vi "Confocal_VerTDVg.vi"() -> ()   [LabVIEW 2009]
uses:
  <vilib>/DAQmx/configure/timing.llb/DAQmx Timing (Sample Clock).vi
  <vilib>/DAQmx/create/channels.llb/DAQmx Create Channel (AI-Voltage-Basic).vi
  <vilib>/DAQmx/create/channels.llb/DAQmx Create Channel (AO-Voltage-Basic).vi
  <vilib>/DAQmx/write.llb/DAQmx Write (Analog 2D DBL NChan NSamp).vi
  <vilib>/DAQmx/read.llb/DAQmx Read (Analog 1D DBL NChan 1Samp).vi
  <vilib>/DAQmx/configure/trigger.llb/DAQmx Start Trigger (Digital Edge).vi
  <vilib>/DAQmx/read.llb/DAQmx Read (Analog 2D DBL NChan NSamp).vi
  <vilib>/DAQmx/write.llb/DAQmx Write (Analog 1D DBL NChan 1Samp).vi
  <vilib>/measure/NI_MABase.lvlib
  Program Files (x86)/National Instruments/LabVIEW 2009/resource/objmgr/daqmx.rc
panel:
  out "Boolean":bool=TRUE
  in  "Update":bool
  in  "StopPoint":dbl
  in  "Concat":bool
  in  "Increment":bool
  in  "stepsize":dbl=0.001
  in  "y 2":cluster{dbl, string, tag}[](array[cluster])=[{1.0, "", "Dev1/ai18"}, {1.0, "", "Dev1/ai16"}, {1.0, "", ""}, {1.0, "", ""}, {0.0, "", ""}, {1.0, "", ""}]
  in  "y":cluster{dbl, string, tag}[](array[cluster])=[{1.0, "", "Dev1/ao1"}, {1.0, "", "Dev1/ao0"}, {1.0, "", "Dev1/ao2"}, {1.0, "", "Dev1/ao3"}, {0.0, "", ""}, {1.0, "", ""}]
  in  "?":bool
  in  "Output4":dbl min=-10.0 max=10.0 step=0.1
  in  "Output3":dbl min=-10.0 max=10.0 step=0.1
  in  "Starting Point for Scan":tag="Dev1/ai1:2"
  in  "output scale":i32=1
  in  "out/in":dbl=1.0
  in  "Channel 2":path=path "C:/Users/debordet/Desktop/Physics Research/CNT PGM/Data/Scans/2011-10-7/J15_[16]_PA1"
  in  "Channel 1":path=path "C:/Users/debordet/Desktop/Physics Research/CNT PGM/Data/Scans/2011-10-7/J15_[16]_Refl1"
  in  "Save Image":bool
  out "Channel2":dbl[][](graph)
  in  "Scanner delay (ms)":dbl=0.16
  in  "Lines read":u32=1
  out "Reflection Image":dbl[][](graph)
  out "Linescan":dbl[][](graph)=[[0.06856738193309811, 0.06824489935784073, 0.06727745163238377, 0.06727745163238377, 0.06792241678263589, 0.06792241678263589, 0.06759993420748357, 0.06792241678263589, 0.06792241678263589, 0.06759993420748357, 0.06792241678263589, 0.06792241678263589, 0.06856738193309811, 0.06792241678263589, 0.06759993420748357, 0.06824489935784073, 0.06759993420748357, 0.06759993420748357, 0.06727745163238377, 0.06727745163238377, 0.06759993420748357, 0.06695496905733647, 0.06759993420748357, 0.06759993420748357, 0.06727745163238377, 0.06856738193309811, 0.06824489935784073, 0.06792241678263589, 0.06792241678263589, 0.06856738193309811, 0.06856738193309811, 0.06856738193309811, 0.06888986450840807, 0.06921234708377061, 0.06985731223465351, 0.06985731223465351, 0.07050227738574695, 0.07050227738574695, 0.07082475996137268, 0.0711472425370511, 0.07146972511278223, 0.07146972511278223, 0.0711472425370511, 0.0711472425370511, 0.07082475996137268, 0.06985731223465351, 0.06985731223465351, 0.06985731223465351, 0.06888986450840807, 0.06824489935784073, 0.06759993420748357, 0.06759993420748357, 0.06727745163238377, 0.06727745163238377, 0.06695496905733647, 0.06695496905733647, 0.06663248648234164, 0.06727745163238377, 0.06695496905733647, 0.06727745163238377, 0.06759993420748357, 0.06759993420748357, 0.06792241678263589, 0.06759993420748357, 0.06856738193309811, 0.06856738193309811, 0.06888986450840807, 0.06792241678263589, 0.06824489935784073, 0.06759993420748357, 0.06792241678263589, 0.06727745163238377, 0.06759993420748357, 0.06695496905733647, 0.06727745163238377, 0.06695496905733647, 0.06663248648234164, 0.06663248648234164, 0.06663248648234164, 0.06631000390739929, 0.06631000390739929, 0.06631000390739929, 0.06631000390739929, 0.06598752133250936, 0.06598752133250936, 0.06566503875767186, 0.06598752133250936, 0.06631000390739929, 0.06598752133250936, 0.06631000390739929, 0.06598752133250936, 0.06534255618288677, 0.06566503875767186, 0.06469759103347372, 0.06437510845884574, 0.06244021301217625, 0.05857042212447406, 0.04825097979380309, 0.04276877607709824, 0.03599664209450654, 0.029546990703332412, 0.025032234741517494, 0.02438726960491914, 0.025677199878316508, 0.02761209528991893, 0.03341678153560791, 0.0401889155096509, 0.04760601464989135, 0.05470063124426199, 0.05953786984569621, 0.062117730437914236, 0.06179524786370443, 0.06308517816085697, 0.06308517816085697, 0.06405262588427009, 0.06502007360815405, 0.06534255618288677, 0.06598752133250936, 0.06534255618288677, 0.06405262588427009, 0.06276269558649049, 0.05953786984569621, 0.05695800925681054, 0.05534559639044516, 0.05405566609828603, 0.05470063124426199, 0.05566807896361449, 0.05502311381732767, 0.053410700952517126, 0.05212077066159994, 0.04857346236583612, 0.04502615407629937, 0.04341374121947115, 0.040511398080403126, 0.040511398080403126, 0.040511398080403126, 0.04147884579296599, 0.0418013283639224, 0.0421238109349299, 0.04276877607709824, 0.0418013283639224, 0.0401889155096509, 0.03760905494546761, 0.03470671181465164, 0.03244933382685677, 0.03180436868794224, 0.03244933382685677, 0.03502919438453927, 0.039221467797700145, 0.04147884579296599, 0.0456711192193894, 0.04792849722182151, 0.04825097979380309, 0.0456711192193894, 0.042446293505988504, 0.03631912466459714, 0.03277181639638989, 0.025032234741517494, 0.02180740906052947, 0.020839961357208617, 0.022129891628403037, 0.02535471730989191, 0.029869473272411, 0.03857650265665441, 0.0456711192193894, 0.05276573580695514, 0.057602974403720045, 0.06115028271544139, 0.06308517816085697, 0.06405262588427009, 0.06598752133250936, 0.06663248648234164, 0.06727745163238377, 0.06727745163238377, 0.06695496905733647, 0.06598752133250936, 0.06534255618288677, 0.06469759103347372, 0.06437510845884574, 0.06373014330974676, 0.06469759103347372, 0.06502007360815405, 0.06566503875767186, 0.06598752133250936, 0.06631000390739929, 0.06566503875767186, 0.06663248648234164, 0.06566503875767186, 0.06534255618288677, 0.06469759103347372, 0.06373014330974676, 0.062117730437914236, 0.060182834993437954, 0.05792545697725274, 0.057602974403720045, 0.056313044110108734, 0.05502311381732767, 0.056313044110108734, 0.05663552668343368, 0.05889290469816274], [0.014390310013197828, 0.01277789718029931, 0.01277789718029931, 0.018260100817215456, 0.017937618249940557, 0.014390310013197828, 0.02180740906052947, 0.02180740906052947, 0.019550031086813136, 0.015035275146704158, 0.021162443924932276, 0.016002722847335796, 0.006328245861055242, 0.011487966914871401, 0.005038315599569377, 0.004070867903970193, 0.013100379746779965, 0.00858562382054782, 0.008908106386386505, 0.012132932047486448, 0.02341982190039753, 0.013745344879889812, 0.03599664209450654, 0.012455414613868144, 0.018582583384540143, 0.01277789718029931, 0.05018587522677358, 0.018582583384540143, 0.018260100817215456, 0.019550031086813136, 0.01406782744651904, 0.01632520541431232, 0.00858562382054782, 0.011487966914871401, 0.008908106386386505, 0.01019803665023418, 0.013745344879889812, 0.01632520541431232, 0.008263141254758391, 0.008263141254758391, 0.008263141254758391, 0.006328245861055242, 0.011487966914871401, 0.015357757713531733, 0.01632520541431232, 0.014390310013197828, 0.021162443924932276, 0.016002722847335796, 0.021484926492705888, 0.013422862313310125, 0.022129891628403037, 0.021162443924932276, 0.016970170548414435, 0.018582583384540143, 0.022774856764300203, 0.016970170548414435, 0.018260100817215456, 0.018582583384540143, 0.01632520541431232, 0.010520519216319421, 0.007295693557685477, 0.00955307151821172, -0.00012140543853553054, 0.004393350469120888, 0.0008460422551557815, 0.006973210992092902, 0.0027809376438573193, 0.007295693557685477, 0.010843001782454027, 0.005683280730214114, 0.022129891628403037, 0.016002722847335796, 0.013745344879889812, 0.026644647583891578, 0.01632520541431232, 0.01277789718029931, 0.009875554084198285, 0.0034259027738158094, 0.009230588952274466, 0.0011685248198171903, 0.014390310013197828, 0.012455414613868144, 0.025677199878316508, 0.019227548519338968, 0.02761209528991893, 0.028257060427522004, -0.01140829516595663, 0.0237423044685213, 0.0421238109349299, 0.014712792579926194, 0.0011685248198171903, 0.02309733933232384, 0.013100379746779965, 0.010520519216319421, 0.0005235596905432037, 0.004393350469120888, 0.007618176123327238, 0.017292653115540065, 0.02309733933232384, 0.018905065951914643, 0.017937618249940557, 0.012455414613868144, 0.013100379746779965, 0.00955307151821172, 0.016002722847335796, 0.017937618249940557, 0.01987251365433717, 0.012132932047486448, 0.01632520541431232, 0.013745344879889812, 0.017292653115540065, 0.013422862313310125, 0.017615135682715433, 0.016647687981338526, 0.018260100817215456, 0.02341982190039753, 0.020839961357208617, 0.024064787036695165, 0.026967130152517085, 0.025032234741517494, 0.02535471730989191, 0.02890202556532645, 0.026644647583891578, 0.02245237419632661, 0.017292653115540065, 0.02341982190039753, 0.02051747878953489, 0.015035275146704158, 0.014712792579926194, 0.012132932047486448, 0.00955307151821172, 0.006650728426549496, 0.01406782744651904, 0.00471583303432061, 0.013100379746779965, 0.01406782744651904, 0.010843001782454027, 0.014712792579926194, 0.019550031086813136, 0.014390310013197828, 0.017292653115540065, 0.013100379746779965, 0.016002722847335796, 0.006650728426549496, 0.011810449481154207, 0.019550031086813136, 0.004393350469120888, 0.017615135682715433, 0.014712792579926194, 0.04696104950618525, 0.016002722847335796, 0.04147884579296599, 0.013745344879889812, 0.011165484348638014, 0.005038315599569377, 0.011165484348638014, 0.015035275146704158, 0.026322165015316323, 0.021162443924932276, 0.01632520541431232, 0.007940658689018203, 0.005038315599569377, 0.013745344879889812, 0.016647687981338526, 0.022129891628403037, 0.02341982190039753, 0.01987251365433717, 0.017615135682715433, 0.010520519216319421, 0.012132932047486448, 0.011165484348638014, 0.00955307151821172, 0.01632520541431232, 0.012132932047486448, 0.007618176123327238, 0.01406782744651904, 0.009875554084198285, 0.01019803665023418, 0.007618176123327238, 0.013100379746779965, 0.010520519216319421, 0.006328245861055242, 0.013745344879889812, 0.006328245861055242, 0.008908106386386505, 0.015035275146704158, 0.013100379746779965, 0.019550031086813136, 0.014712792579926194, 0.018582583384540143, 0.01987251365433717, 0.011810449481154207, 0.013100379746779965, 0.015035275146704158, 0.017615135682715433, 0.010843001782454027, 0.00858562382054782, 0.006973210992092902, 0.01019803665023418, 0.007618176123327238]]
  out "Output rate":dbl=31250.0
  out "Input rate":dbl=31250.0
  in  "Y Scan size(um)":dbl=3.0
  in  "Reset":bool
  in  "Stop":bool
  in  "Continuous \nScan":bool=TRUE
  in  "Finite scan":bool
  in  "Conversion \n(mV/um)":dbl=41.0
  in  "Scan Lines":u32=200
  in  "Scan Points":u32=200
  in  "Scan Angle (degrees)":dbl
  in  "X offset (um)":dbl
  in  "Y offset (um)":dbl
  in  "Scan Rate (Hz)":dbl=25.0
  in  "X Scan size(um)":dbl=3.0
  in  "minimum value":dbl=-4.0 caption="Output Minimum Value" format="%0.2f"
  in  "maximum value":dbl=4.0 caption="Output Maximum Value" format="%0.2f"
  in  "Maximum Value":dbl=10.0 caption="Input Maximum Value" format="%0.2f"
  in  "Minimum Value":dbl=-10.0 caption="Input Minimum Value" format="%0.2f"
  # "Scan channel 1"
  # "Scan channel 2"
  # "Device"
  # "Output channel 3"
  # "Output channel 4"
  # "Input channel 1"
  # "Input channel 2"
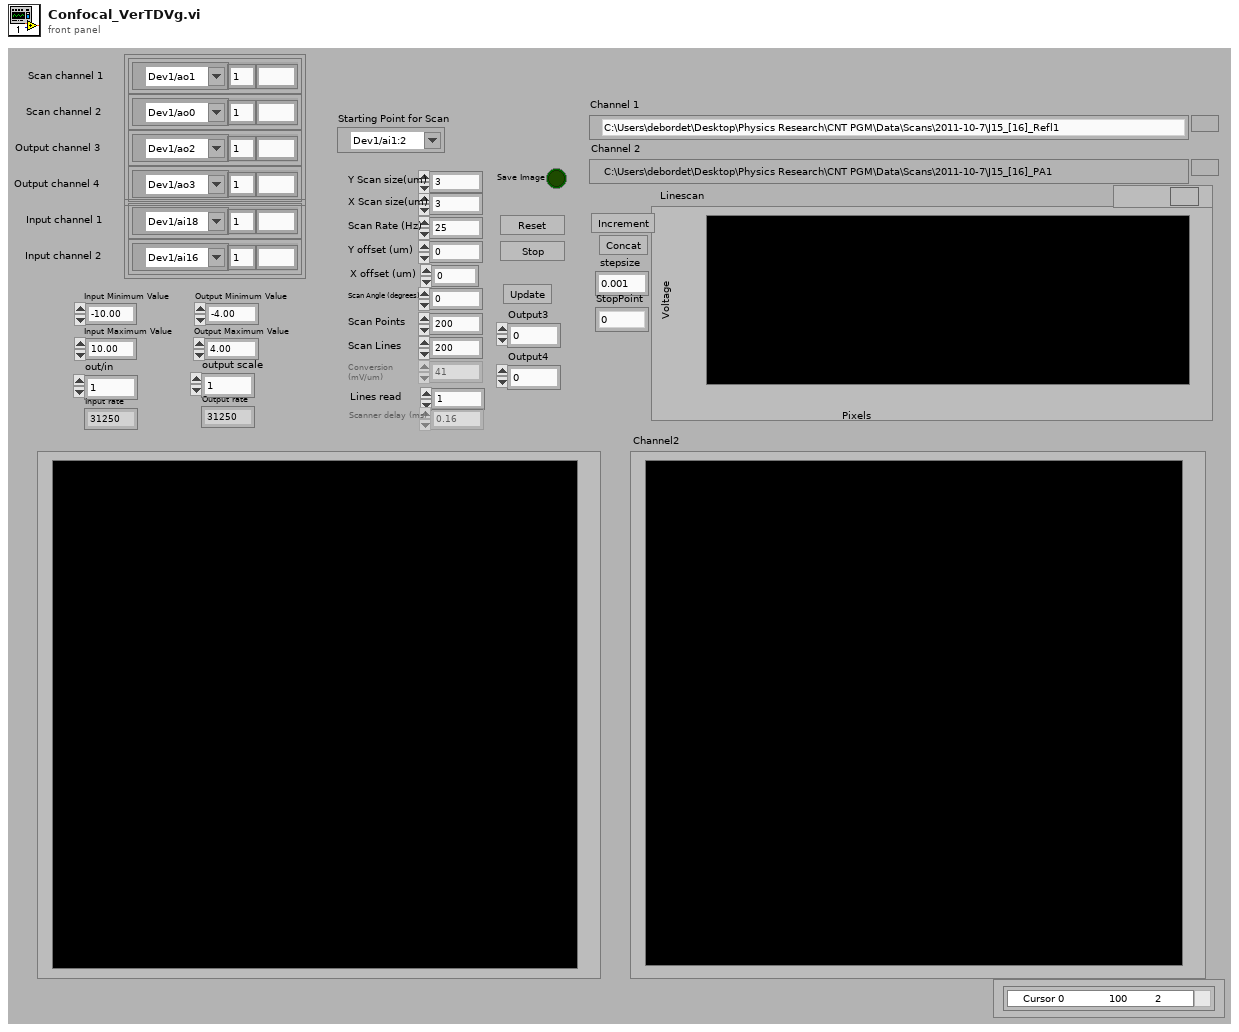
[diagram p1: front panel]
types:
  T1 = enum16{"Sine Wave", "Triangle Wave", "Square Wave", "Sawtooth Wave"}
  T2 = cluster{"Y Scan size(um) ":dbl, "X Scan size(um)":dbl, "Scan Rate (Hz)":dbl, "Y offset (um)":dbl, "X offset (um)":dbl, "Scan Angle (degrees)":dbl, "Scan Points":u32, "Scan Lines":u32, "Conversion \n(mV/um)":dbl, "Finite scan":bool, "Continuous \nScan":bool, "Lines read":u32, "Scanner delay (ms)":dbl}
  T3 = enum16{"open", "open or create", "create or replace", "create", "open (read only)"}
  T4 = typedef "LVPointDoubleTypeDef.ctl" = cluster{"Cursor X":dbl, "Cursor Y":dbl}
  T5 = cluster{"X offset (um)":dbl, "Y offset (um)":dbl}
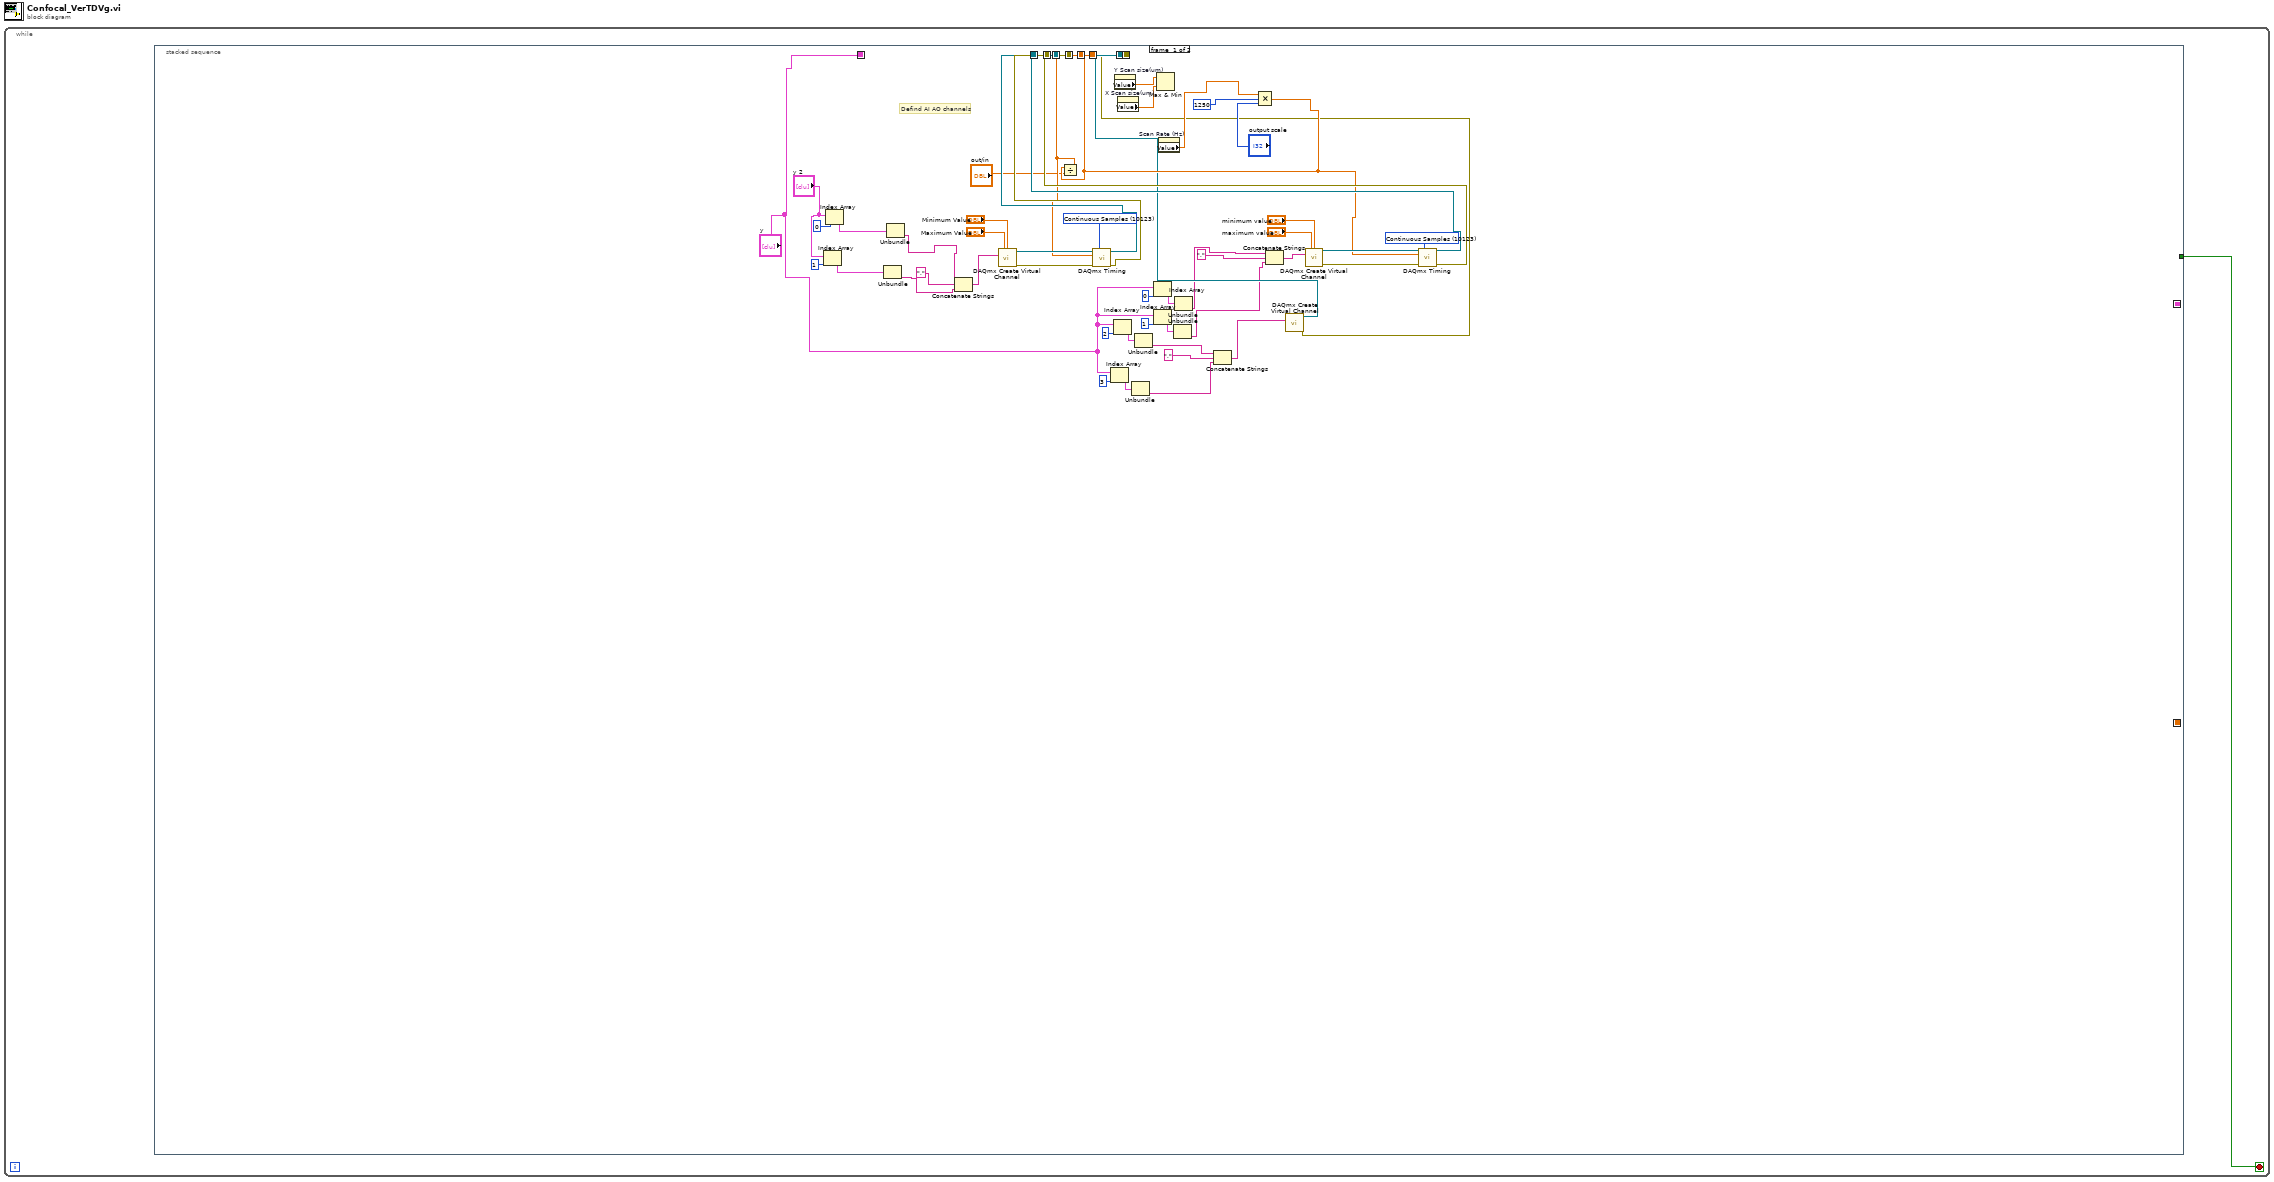
[diagram p0: block diagram]
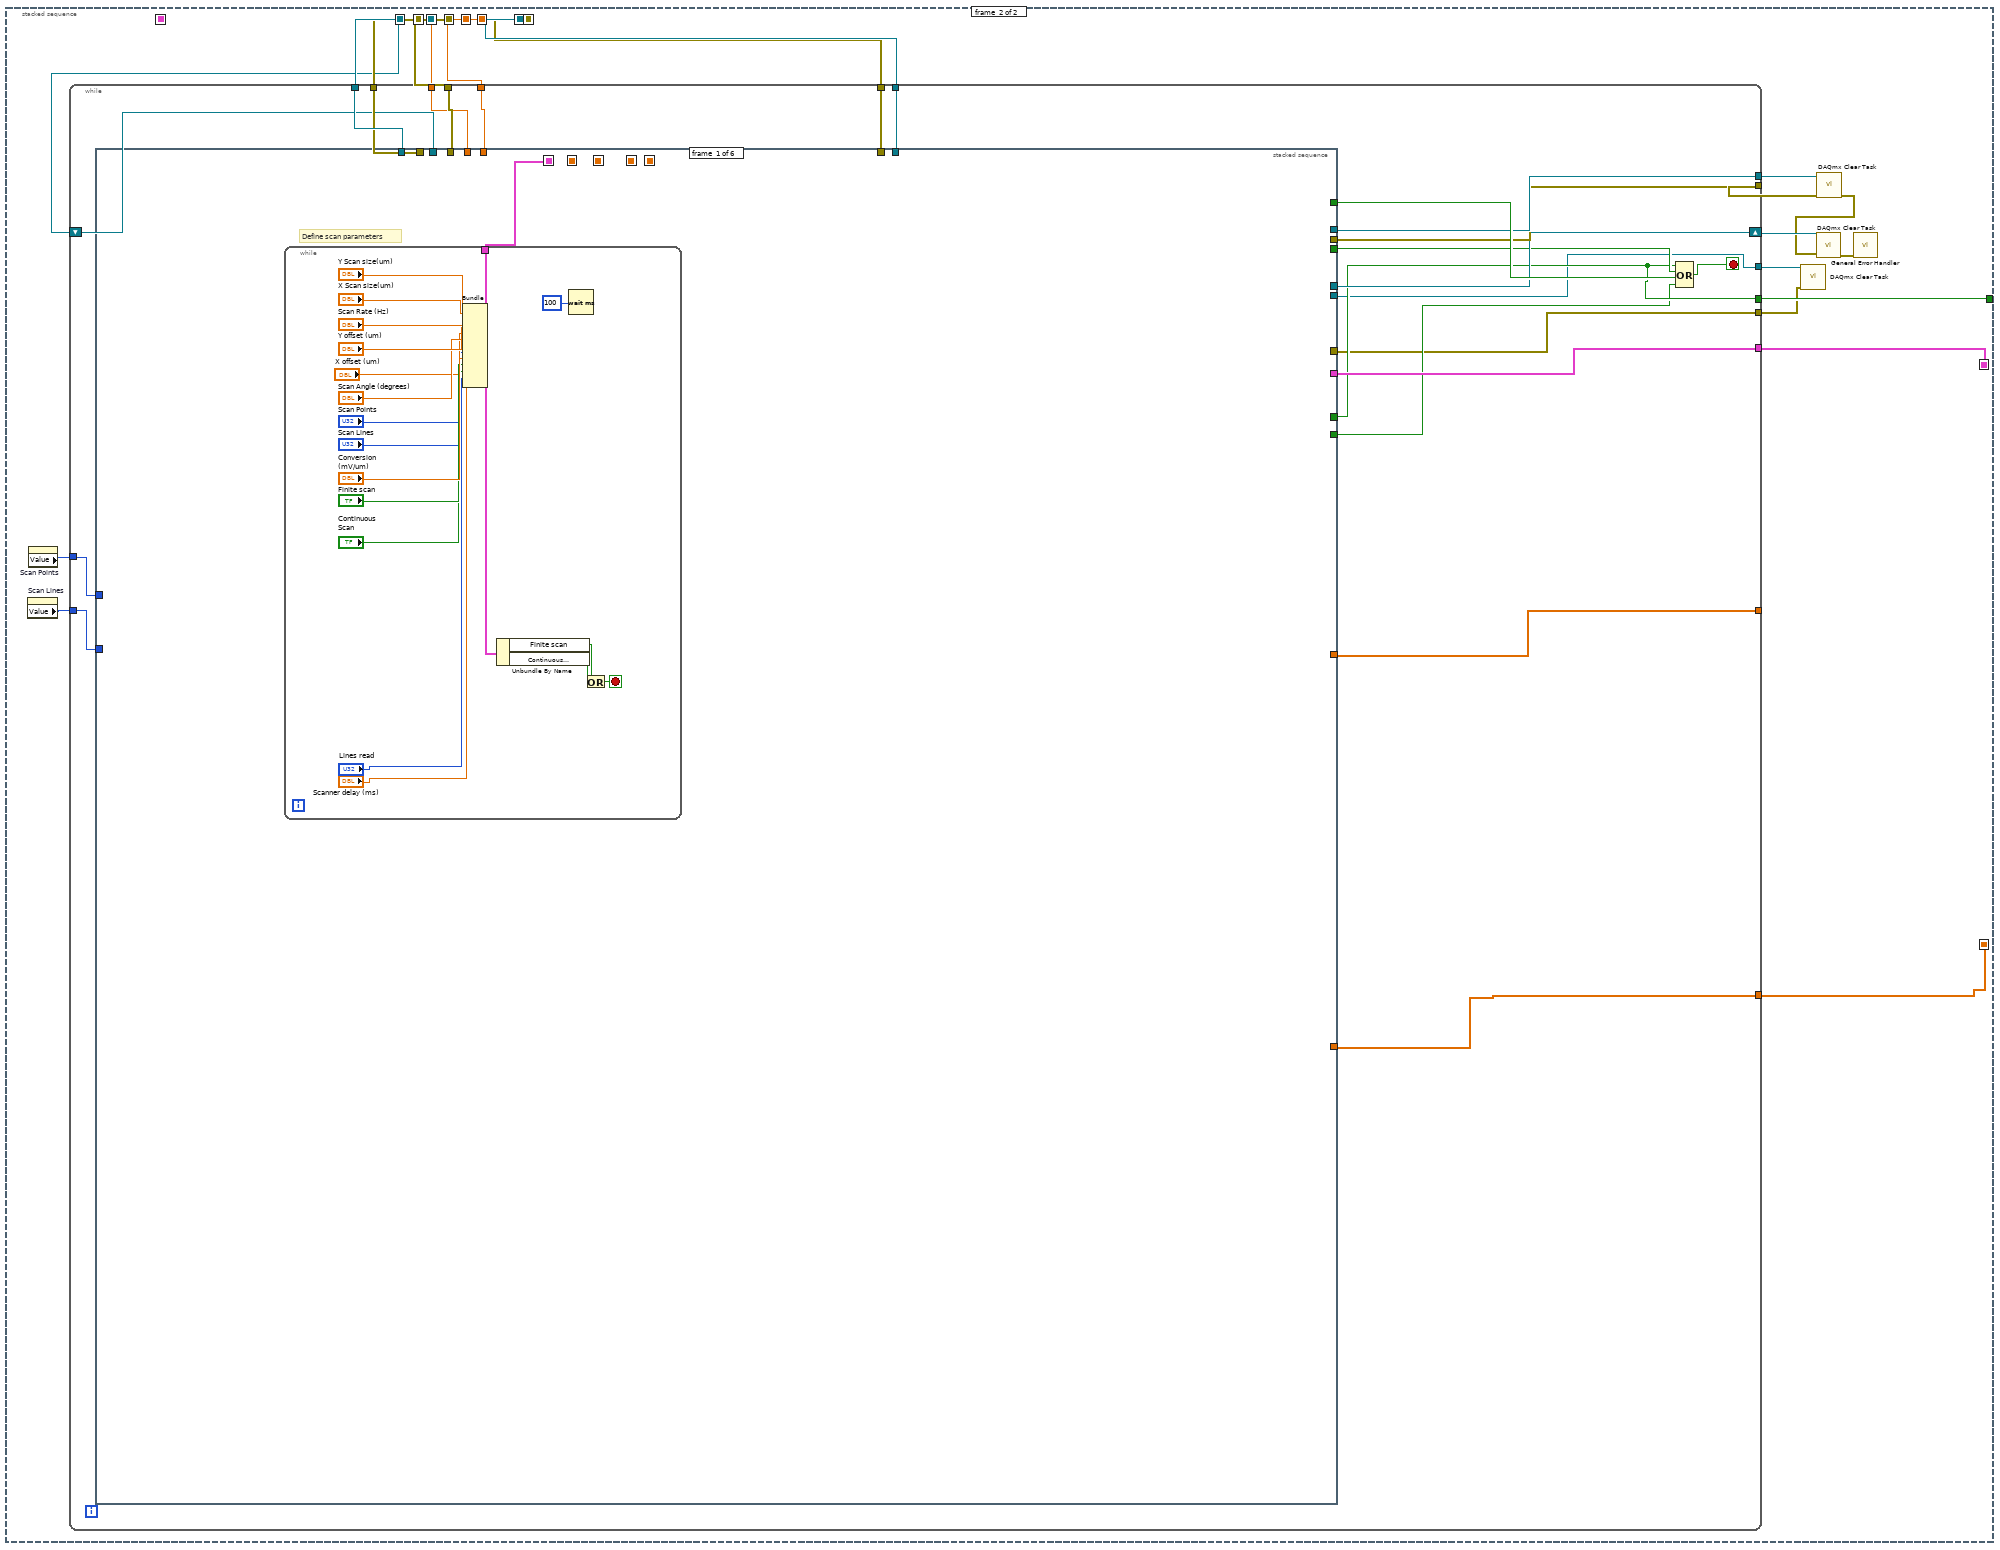
[diagram p2: hidden frame]
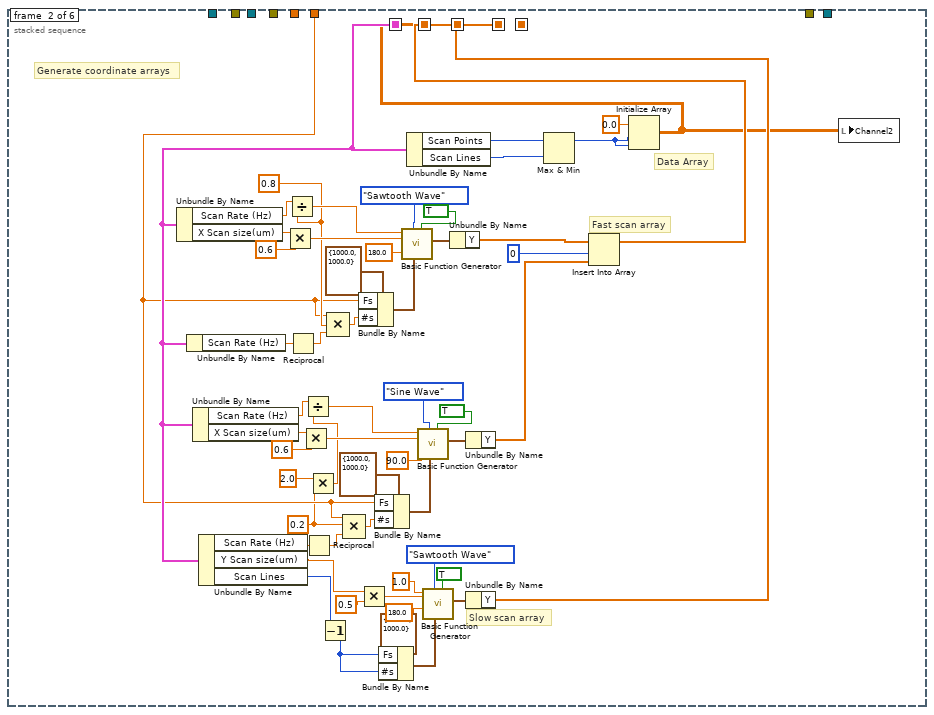
[diagram p3: hidden frame]
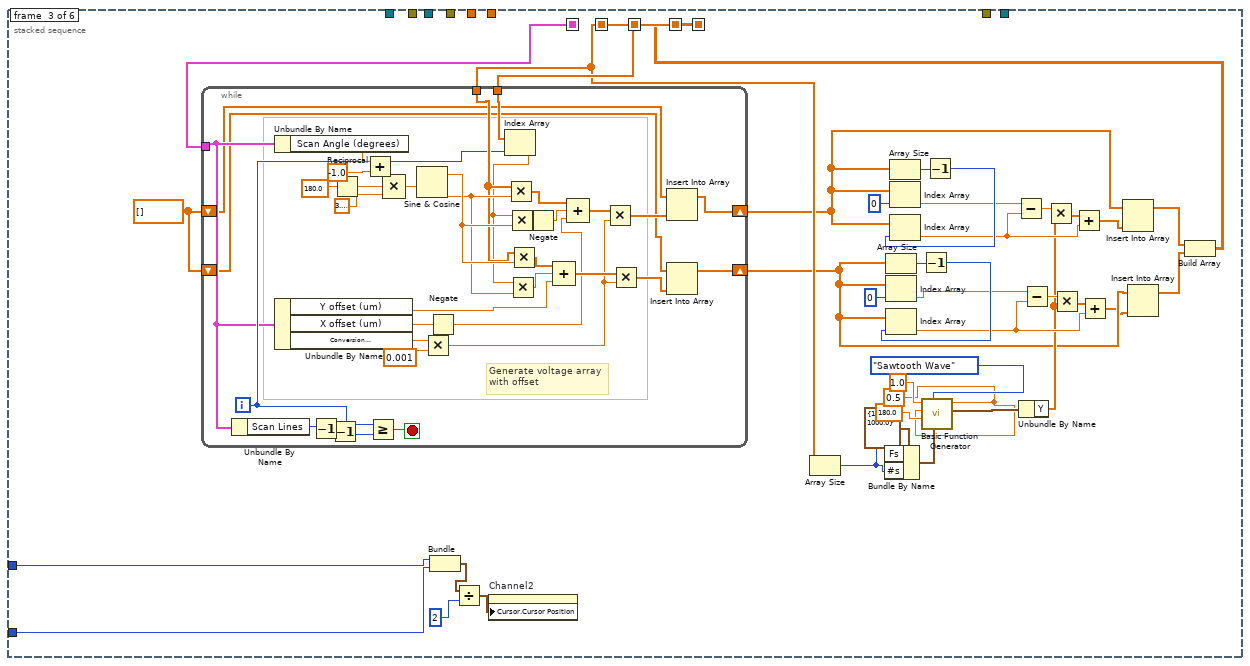
[diagram p4: hidden frame]
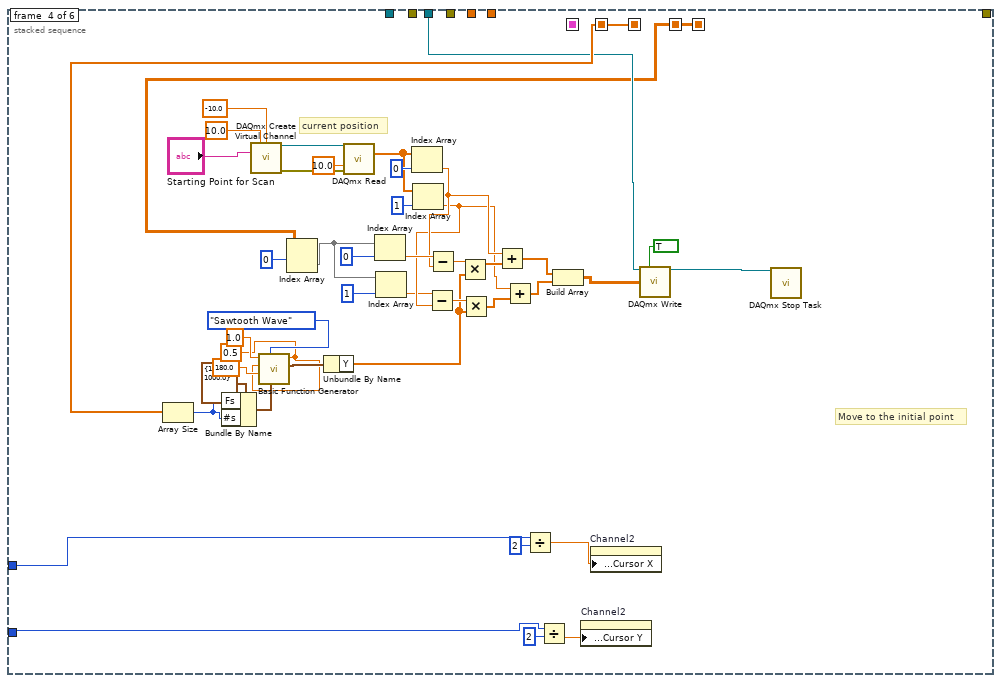
[diagram p5: hidden frame]
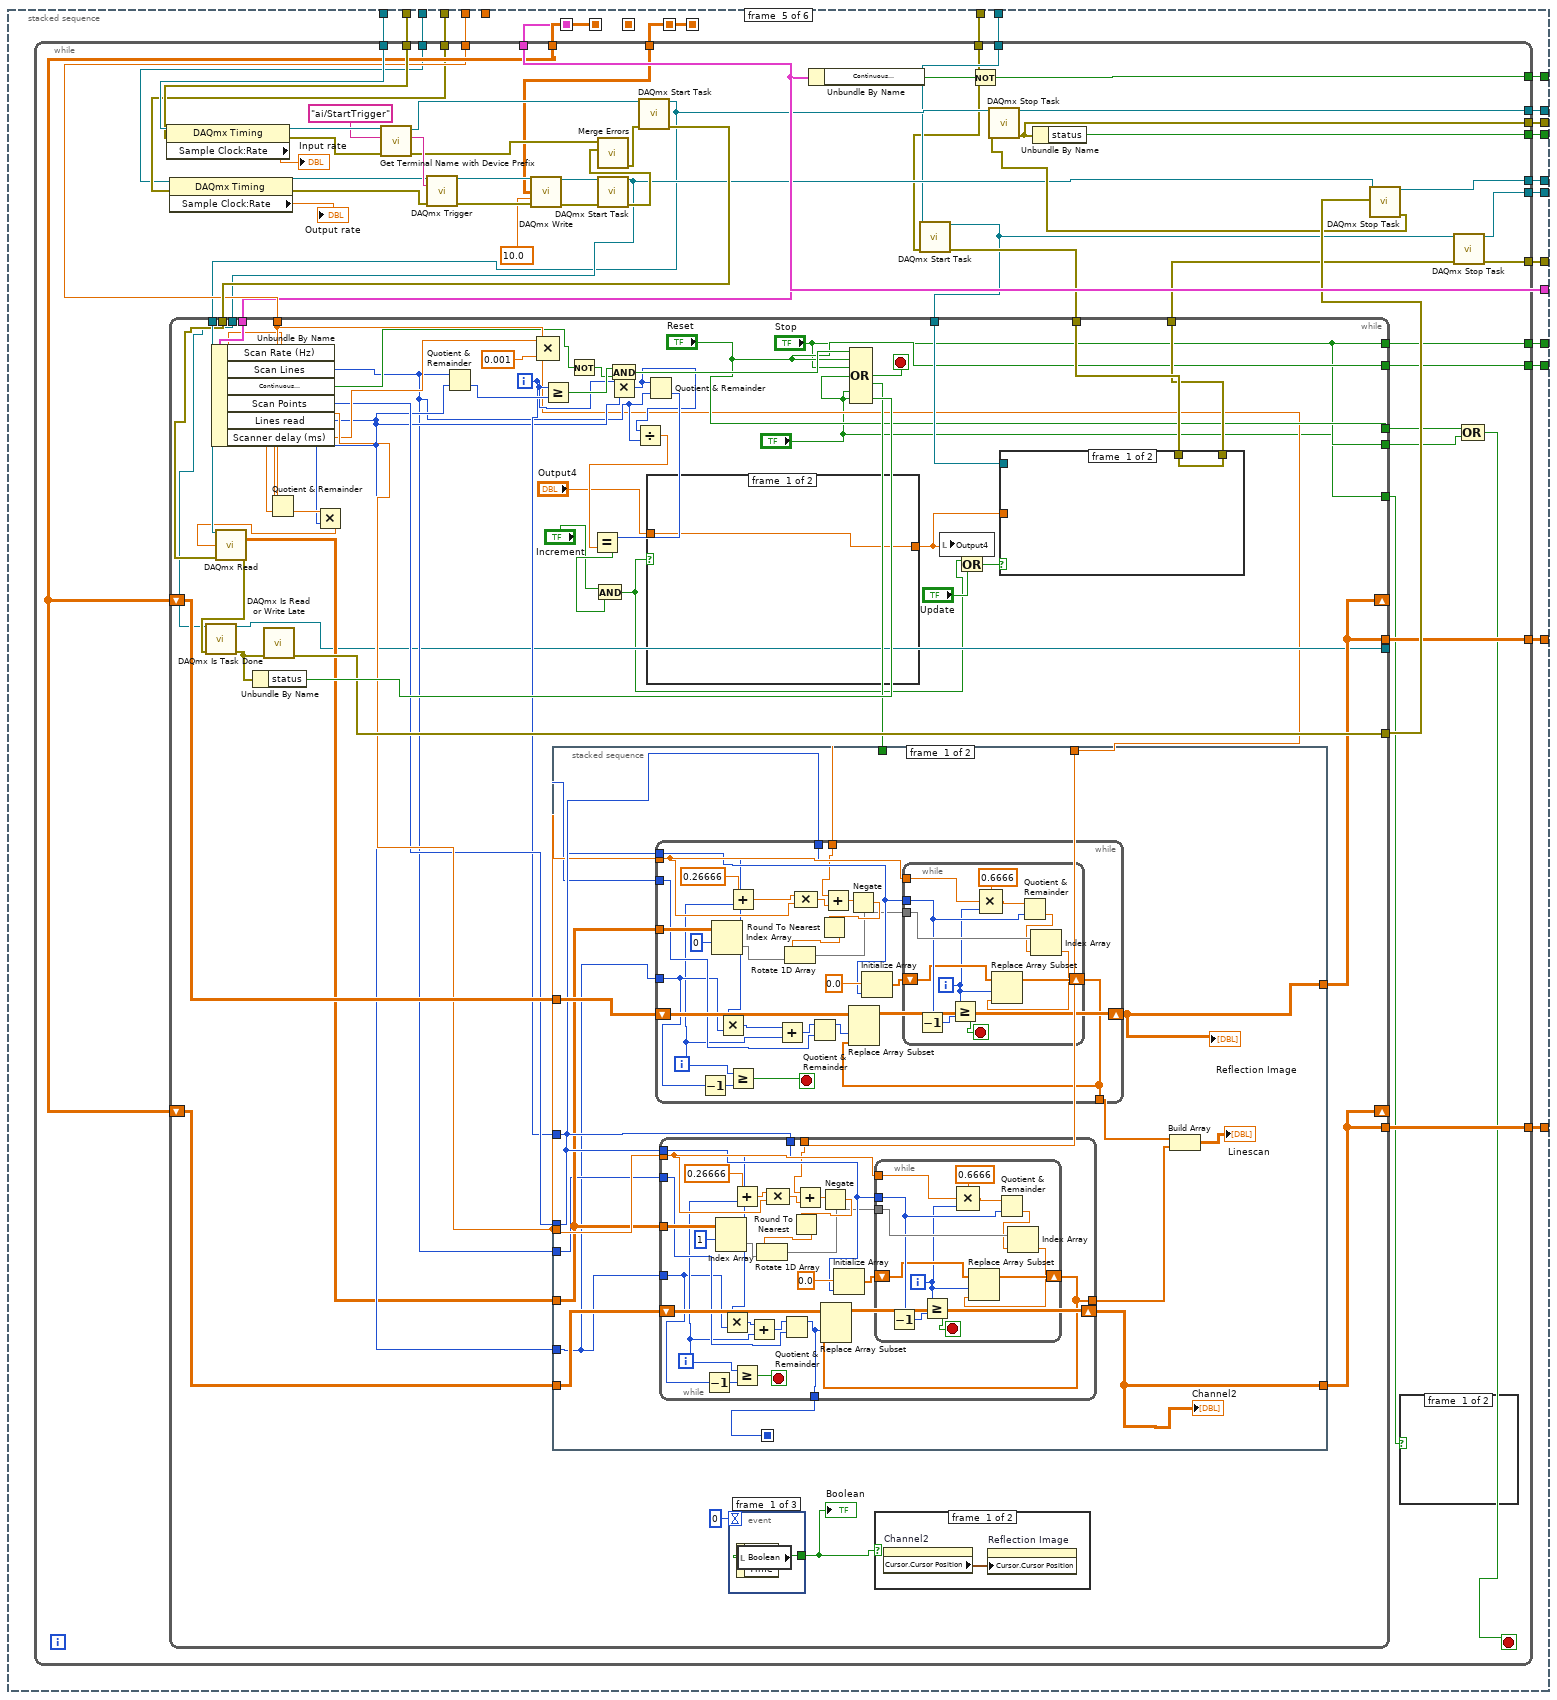
[diagram p6: hidden frame]
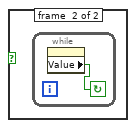
[diagram p7: hidden frame]
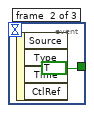
[diagram p8: hidden frame]
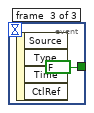
[diagram p9: hidden frame]
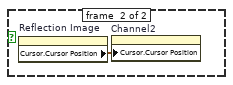
[diagram p10: hidden frame]
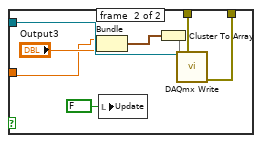
[diagram p11: hidden frame]
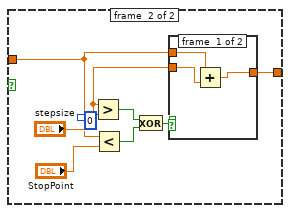
[diagram p12: hidden frame]
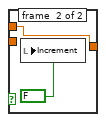
[diagram p13: hidden frame]
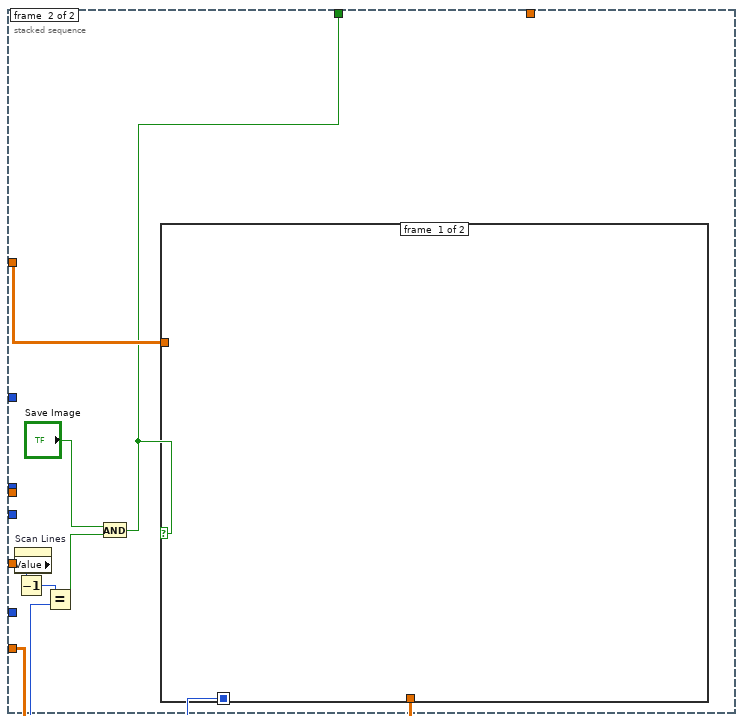
[diagram p14: hidden frame]
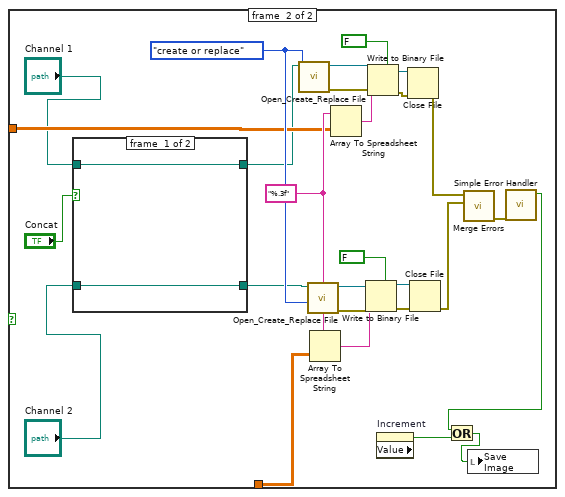
[diagram p15: hidden frame]
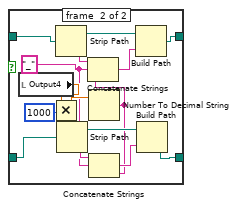
[diagram p16: hidden frame]
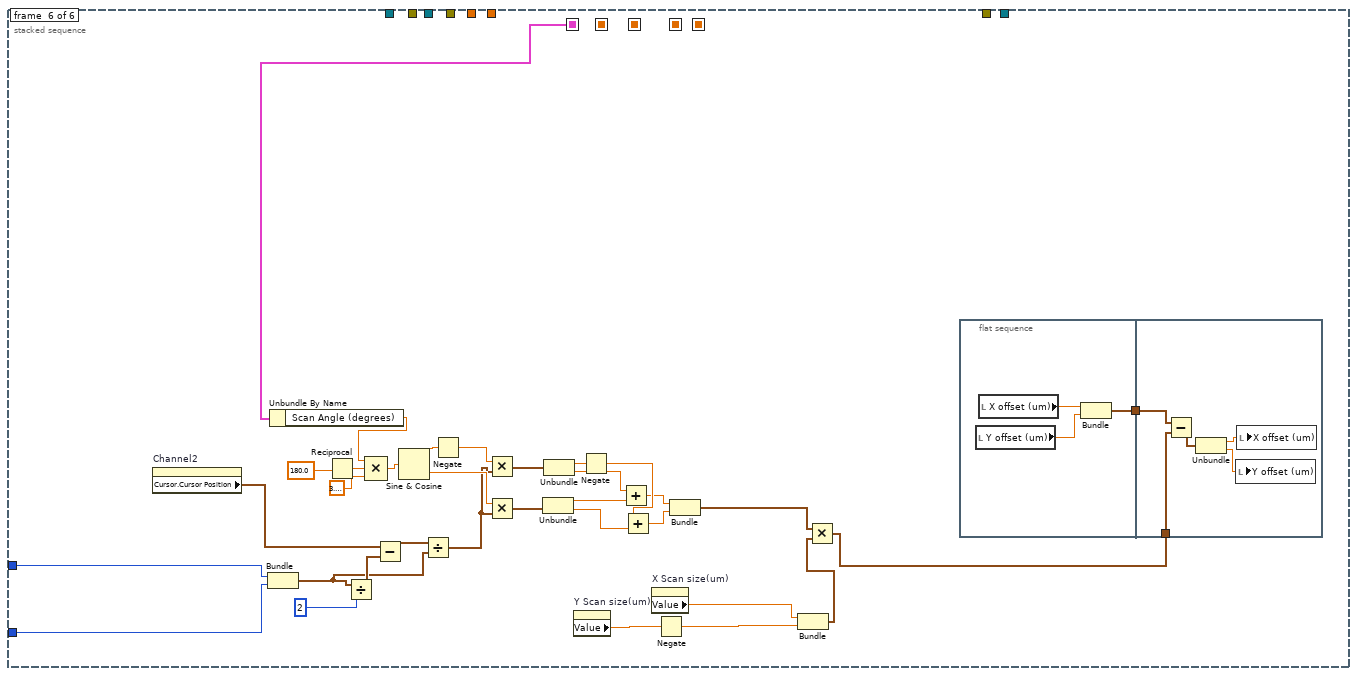
[diagram p17: hidden frame]
diagram:
  n1 = while {
    stop <- w1 stop-if-true
    n2 = stacked-sequence {
      seq-local: [w39 _] -> [_ w70]
      seq-local: [w42 _] -> [_ w69]
      seq-local: [w41 _] -> [_ w62]
      seq-local: [w40 _] -> [_ w68]
      seq-local: [w34 _] -> [_ w67]
      seq-local: [w33 _] -> [_ w71]
      seq-local: [_ w61] -> [_ _]
      seq-local: [_ w60] -> [_ _]
      seq-local: [w29 _] -> [_ w56]
      seq-local: [w28 _] -> [_ w55]
      seq-local: ["y" _] -> [_ _]
      tunnel: [_ w57] -> w1
      frame #0 {
        w44 = 10123 items=["Finite Samples"=10178, "Continuous Samples"=10123] ("sample mode")
        w49 = 10123 items=["Finite Samples"=10178, "Continuous Samples"=10123] ("sample mode")
        # "Defind AI AO channels"
        n3 = Index Array(array="y 2", index=1) -> (element=w20:cluster{dbl, string, tag})
        n4 = Index Array(array="y 2", index=0) -> (element=w22:cluster{dbl, string, tag})
        n5 = Unbundle(w20) -> (w2:tag)  [unwired: 2 out]
        n6 = Unbundle(w22) -> (w3:tag)  [unwired: 2 out]
        n7 = Concatenate Strings(w3, ",", w2) -> (w27:string)
        n8 = call-poly <vilib>:"DAQmx Create Virtual Channel.vi"("maximum value"="Maximum Value", "minimum value"="Minimum Value", "physical channels"=w27) -> ("task out"=w47:refnum<k21>, "error out"=w48:errorcluster)  [unwired: 11 in]
        n9 = Index Array(array="y", index=3) -> (element=w15:cluster{dbl, string, tag})
        n10 = Index Array(array="y", index=2) -> (element=w17:cluster{dbl, string, tag})
        n11 = property on="Y Scan size(um)" class="Digital (strict)"() -> ("Value"=w36:dbl)  [unwired: 2 in, 2 out]
        n12 = property on="X Scan size(um)" class="Digital (strict)"() -> ("Value"=w35:dbl)  [unwired: 2 in, 2 out]
        n13 = Unbundle(w15) -> (w13:tag)  [unwired: 2 out]
        n14 = Unbundle(w17) -> (w14:tag)  [unwired: 2 out]
        n15 = Index Array(array="y", index=1) -> (element=w9:cluster{dbl, string, tag})
        n16 = Index Array(array="y", index=0) -> (element=w11:cluster{dbl, string, tag})
        n17 = Max & Min(x=w36, y=w35) -> ()  [unwired: 2 out]
        n18 = property on="Scan Rate (Hz)" class="Digital (strict)"() -> ("Value"=w31:dbl)  [unwired: 2 in, 2 out]
        n19 = Unbundle(w9) -> (w7:tag)  [unwired: 2 out]
        n20 = Unbundle(w11) -> (w8:tag)  [unwired: 2 out]
        n21 = Concatenate Strings(w14, ",", w13) -> (w4:string)
        n22 = Compound Arithmetic op=MULTIPLY(w31, 1250, "output scale") -> (w33:dbl)
        n23 = Divide(x=w33, y="out/in") -> (x/y=w34:dbl)
        n24 = call-poly <vilib>:"DAQmx Timing.vi"("task/channels in"=w47, "sample mode"=w49, "rate"=w34, "error in"=w48) -> ("task out"=w39:refnum<k21>, "error out"=w42:errorcluster)  [unwired: 10 in]
        n25 = Concatenate Strings(w8, ",", w7) -> (w24:string)
        n26 = call-poly <vilib>:"DAQmx Create Virtual Channel.vi"("physical channels"=w4) -> ("task out"=w29:refnum<k21>, "error out"=w28:errorcluster)  [unwired: 13 in]
        n27 = call-poly <vilib>:"DAQmx Create Virtual Channel.vi"("maximum value"="maximum value", "minimum value"="minimum value", "physical channels"=w24) -> ("task out"=w38:refnum<k21>, "error out"=w43:errorcluster)  [unwired: 11 in]
        n28 = call-poly <vilib>:"DAQmx Timing.vi"("task/channels in"=w38, "sample mode"=w44, "rate"=w33, "error in"=w43) -> ("task out"=w41:refnum<k21>, "error out"=w40:errorcluster)  [unwired: 10 in]
      }
      frame #1 {
        n29 = property on="Scan Lines" class="Digital (strict)"() -> ("Value"=w59:u32)  [unwired: 2 in, 2 out]
        n30 = property on="Scan Points" class="Digital (strict)"() -> ("Value"=w58:u32)  [unwired: 2 in, 2 out]
        n31 = while {
          tunnel: w71 -> [w94]
          tunnel: w70 -> [w93]
          tunnel: w69 -> [w92]
          tunnel: w68 -> [w91]
          tunnel: w67 -> [w90]
          tunnel: [w88] -> w66
          tunnel: [w87] -> w65
          shift-right: [w85] -> w64
          shift-left: w62 -> [w84]
          tunnel: [w83] -> _
          tunnel: [w82] -> w61
          tunnel: [w80] -> w60
          tunnel: w59 -> [w79]
          tunnel: w58 -> [w78]
          tunnel: [w77] -> w57
          tunnel: w56 -> [w75]
          tunnel: w55 -> [w74]
          tunnel: [w73] -> w53
          tunnel: [w72] -> w52
          stop <- w86 stop-if-true
          n32 = stacked-sequence {
            seq-local: [w95 _ _ _ _ _] -> [_ w139 w207 _ w295 w612]
            seq-local: [_ w114 _ _ _ _] -> [_ _ _ _ w302 _]
            seq-local: [_ w115 _ _ _ _] -> [_ _ w197 w256 _ _]
            seq-local: [_ w116 _ _ _ _] -> [_ _ w208 _ _ _]
            seq-local: [_ _ w170 _ _ _] -> [_ _ _ w252 w299 _]
            tunnel: w94 -> [_ w138 _ _ _ _]
            tunnel: w93 -> [_ _ _ _ w310 _]
            tunnel: w92 -> [_ _ _ _ w309 _]
            tunnel: w84 -> [_ _ _ w254 w298 _]
            tunnel: w91 -> [_ _ _ _ w308 _]
            tunnel: w90 -> [_ _ _ _ w300 _]
            tunnel: [_ _ _ _ w307 _] -> w77
            tunnel: [_ _ _ _ w306 _] -> w81
            tunnel: [_ _ _ _ w301 _] -> w89
            tunnel: [_ _ _ _ w305 _] -> w88
            tunnel: [_ _ _ _ w304 _] -> w87
            tunnel: [_ _ _ _ w303 _] -> w85
            tunnel: [_ _ _ _ w297 _] -> w83
            tunnel: [_ _ _ _ w296 _] -> w82
            tunnel: [_ _ _ _ w295 _] -> w80
            tunnel: [_ _ _ _ w294 _] -> w76
            tunnel: w79 -> [_ _ w172 w246 _ w587]
            tunnel: w78 -> [_ _ w173 w247 _ w586]
            tunnel: w75 -> [_ _ _ _ w293 _]
            tunnel: w74 -> [_ _ _ _ w292 _]
            tunnel: [_ _ _ _ w291 _] -> w73
            tunnel: [_ _ _ _ w290 _] -> w72
            frame #0 {
              # "Define scan parameters"
              n33 = while {
                tunnel: [w106] -> w95
                stop <- w107 stop-if-true
                n34 = Bundle("Y Scan size(um)"="Y Scan size(um)", "X Scan size(um)"="X Scan size(um)", "Scan Rate (Hz)"="Scan Rate (Hz)", "Y offset (um)"="Y offset (um)", "X offset (um)"="X offset (um)", "Scan Angle (degrees)"="Scan Angle (degrees)", "Scan Points"="Scan Points", "Scan Lines"="Scan Lines", "Conversion \n(mV/um)"="Conversion \n(mV/um)", "Finite scan"="Finite scan", "Continuous \nScan"="Continuous \nScan", "Lines read"="Lines read", "Scanner delay (ms)"="Scanner delay (ms)") -> (w106:T2)  [unwired: 1 in]
                n35 = Unbundle By Name(w106) -> ("Finite scan"=w105:bool, "Continuous \nScan"=w104:bool)
                n36 = Wait (ms)(milliseconds to wait=u32 100) -> ()  [unwired: 1 out]
                n37 = Or(x=w105, y=w104) -> (x .or. y?=w107:bool)
              }
            }
            frame #1 {
              w118 = 0.2 ("value")
              w157 = 0.8 ("y")
              # "Slow scan array"
              # "Fast scan array"
              # "Data Array"
              # "Generate coordinate arrays"
              n38 = Unbundle By Name(w139) -> ("Scan Rate (Hz)"=w162:dbl, "X Scan size(um)"=w165:dbl)
              n39 = Unbundle By Name(w139) -> ("Scan Rate (Hz)"=w155:dbl)
              n40 = Unbundle By Name(w139) -> ("Scan Rate (Hz)"=w147:dbl, "X Scan size(um)"=w150:dbl)
              n41 = Unbundle By Name(w139) -> ("Scan Rate (Hz)"=w141:dbl, "Y Scan size(um)"=w130:dbl, "Scan Lines"=w131:u32)
              n42 = Multiply(x=w165, y=0.6) -> (x*y=w163:dbl)
              n43 = Divide(x=w162, y=w157) -> (x/y=w161:dbl)
              n44 = Reciprocal(x=w155) -> (1/x=w156:dbl)
              n45 = Multiply(x=w150, y=0.6) -> (x*y=w148:dbl)
              n46 = Reciprocal(x=w141) -> (1/x=w142:dbl)
              n47 = Multiply(x=2.0, y=w118) -> (x*y=w117:dbl)
              n48 = Divide(x=w147, y=w117) -> (x/y=w146:dbl)
              n49 = Decrement(x=w131) -> (x-1=w123:u32)
              n50 = Compound Arithmetic op=MULTIPLY(w138, w157, w156) -> (w158:dbl)
              n51 = Compound Arithmetic op=MULTIPLY(w138, w118, w142) -> (w143:dbl)
              n52 = Bundle By Name(cluster=cluster{"Fs":dbl, "#s":dbl} {"Fs"=1000.0, "#s"=1000.0} ("sampling info"), "Fs"=w138, "#s"=w158) -> (w159:cluster{"Fs":dbl, "#s":dbl})
              n53 = Multiply(x=w130, y=0.5) -> (x*y=w129:dbl)
              n54 = Bundle By Name(cluster=cluster{"Fs":dbl, "#s":dbl} {"Fs"=1000.0, "#s"=1000.0} ("sampling info"), "Fs"=w138, "#s"=w143) -> (w144:cluster{"Fs":dbl, "#s":dbl})
              n55 = Bundle By Name(cluster=cluster{"Fs":dbl, "#s":dbl} {"Fs"=1000.0, "#s"=1000.0} ("sampling info"), "Fs"=w123, "#s"=w123) -> (w132:cluster{"Fs":dbl, "#s":dbl})
              n56 = call <vilib>:"Basic Function Generator.vi"("reset signal"=TRUE, "sampling info"=w159, "signal type"=T1."Sawtooth Wave", "phase"=180.0, "amplitude"=w163, "frequency"=w161) -> ("signal out"=w154:waveform(dbl))  [unwired: 3 in, 2 out]
              n57 = Unbundle By Name(w139) -> ("Scan Points"=w122:u32, "Scan Lines"=w121:u32)
              n58 = call <vilib>:"Basic Function Generator.vi"("reset signal"=TRUE, "sampling info"=w144, "signal type"=T1."Sine Wave", "phase"=90.0, "amplitude"=w148, "frequency"=w146) -> ("signal out"=w140:waveform(dbl))  [unwired: 3 in, 2 out]
              n59 = call <vilib>:"Basic Function Generator.vi"("reset signal"=TRUE, "sampling info"=w132, "signal type"=T1."Sawtooth Wave", "phase"=180.0, "amplitude"=w129, "frequency"=1.0) -> ("signal out"=w125:waveform(dbl))  [unwired: 3 in, 2 out]
              n60 = Unbundle By Name(w154) -> ("Y"=w127:dbl[])
              n61 = Unbundle By Name(w140) -> ("Y"=w137:dbl[])
              n62 = Unbundle By Name(w125) -> ("Y"=w116:dbl[])
              n63 = Max & Min(x=w122, y=w121) -> (max(x,y)=w120:u32)  [unwired: 1 out]
              n64 = Insert Into Array(array=w127, index=0, new element=w137) -> (w115:dbl[])
              n65 = Initialize Array(0.0 ("element"), w120, w120) -> (w114:dbl[][])
              n66 = local write "Channel2"(w114) -> ()
            }
            frame #2 {
              w199 = 0.5 ("offset")
              w206 = dbl[] []
              n67 = while {
                tunnel: w207 -> [w228]
                tunnel: w197 -> [w234]
                tunnel: w208 -> [w233]
                shift-right: [w220] -> w179
                shift-left: w206 -> [w219]
                shift-right: [w216] -> w180
                shift-left: w206 -> [w217]
                i -> [w231]
                stop <- w225 stop-if-true
                # "Generate voltage array\nwith offset"
                n68 = Unbundle By Name(w228) -> ("Scan Lines"=w230:u32)
                n69 = Unbundle By Name(w228) -> ("Scan Angle (degrees)"=w244:dbl)
                n70 = Unbundle By Name(w228) -> ("Y offset (um)"=w209:dbl, "X offset (um)"=w211:dbl, "Conversion \n(mV/um)"=w227:dbl)
                n71 = Decrement(x=w230) -> (x-1=w229:u32)
                n72 = Decrement(x=w229) -> (x-1=w215:u32)
                n73 = Reciprocal(x=180.0 ("value")) -> (1/x=w243:dbl)
                n74 = Add(x=w244, y=-1.0) -> (x+y=w214:dbl)
                n75 = Greater Or Equal?(x=w231, y=w215) -> (x >= y?=w225:bool)
                n76 = Compound Arithmetic op=MULTIPLY(w214, w243, 3.141592653589793) -> (w245:dbl)
                n77 = Sine & Cosine(0:w245) -> (1:w241:dbl, 2:w240:dbl)
                n78 = Multiply(x=w227, y=0.001) -> (x*y=w222:dbl)
                n79 = Negate(x=w211) -> (-x=w210:dbl)
                n80 = Index Array(array=w233, index=w231) -> (element=w232:dbl)
                n81 = Multiply(x=w234, y=w240) -> (x*y=w237:dbl[])
                n82 = Multiply(x=w232, y=w241) -> (x*y=w239:dbl)
                n83 = Multiply(x=w232, y=w240) -> (x*y=w236:dbl)
                n84 = Multiply(x=w234, y=w241) -> (x*y=w235:dbl[])
                n85 = Negate(x=w239) -> (-x=w238:dbl)
                n86 = Compound Arithmetic op=unknown(w235, w236, w209) -> (w223:dbl[])
                n87 = Compound Arithmetic op=unknown(w237, w238, w210) -> (w224:dbl[])
                n88 = Multiply(x=w224, y=w222) -> (x*y=w221:dbl[])
                n89 = Multiply(x=w223, y=w222) -> (x*y=w218:dbl[])
                n90 = Insert Into Array(array=w219, new element=w221) -> (w220:dbl[])  [unwired: 1 in]
                n91 = Insert Into Array(array=w217, new element=w218) -> (w216:dbl[])  [unwired: 1 in]
              }
              n92 = Bundle("Value"=w173, "Value"=w172) -> (w171:cluster{"Value":u32, "Value":u32})  [unwired: 1 in]
              n93 = Divide(x=w171, y=2) -> (x/y=w175:cluster{"Value":dbl, "Value":dbl})
              n94 = property on="Channel2" class="IntensityGraph (strict)"("Cursor.Cursor Position"=w175) -> ()  [unwired: 2 in, 2 out]
              n95 = Array Size(array=w197) -> (size(s)=w198:i32)
              n96 = Bundle By Name(cluster=cluster{"Fs":dbl, "#s":dbl} {"Fs"=1000.0, "#s"=1000.0} ("sampling info"), "Fs"=w198, "#s"=w198) -> (w203:cluster{"Fs":dbl, "#s":dbl})
              n97 = Array Size(array=w180) -> (size(s)=w192:i32)
              n98 = Index Array(array=w180, index=0) -> (element=w184:dbl)
              n99 = Array Size(array=w179) -> (size(s)=w195:i32)
              n100 = Index Array(array=w179, index=0) -> (element=w189:dbl)
              n101 = Decrement(x=w192) -> (x-1=w191:i32)
              n102 = Index Array(array=w180, index=w191) -> (element=w183:dbl)
              n103 = call <vilib>:"Basic Function Generator.vi"("offset"=w199, "sampling info"=w203, "signal type"=T1."Sawtooth Wave", "phase"=180.0, "amplitude"=w199, "frequency"=1.0) -> ("signal out"=w201:waveform(dbl))  [unwired: 3 in, 2 out]
              n104 = Decrement(x=w195) -> (x-1=w194:i32)
              n105 = Index Array(array=w179, index=w194) -> (element=w187:dbl)
              n106 = Subtract(x=w189, y=w187) -> (x-y=w190:dbl)
              n107 = Unbundle By Name(w201) -> ("Y"=w182:dbl[])
              n108 = Subtract(x=w184, y=w183) -> (x-y=w186:dbl)
              n109 = Multiply(x=w190, y=w182) -> (x*y=w188:dbl[])
              n110 = Multiply(x=w186, y=w182) -> (x*y=w185:dbl[])
              n111 = Add(x=w188, y=w187) -> (x+y=w181:dbl[])
              n112 = Add(x=w185, y=w183) -> (x+y=w176:dbl[])
              n113 = Insert Into Array(array=w179, new element=w181) -> (w178:dbl[])  [unwired: 1 in]
              n114 = Insert Into Array(array=w180, new element=w176) -> (w177:dbl[])  [unwired: 1 in]
              n115 = Build Array(w178, w177) -> (w170:dbl[][])
            }
            frame #3 {
              w276 = 0.5 ("offset")
              # "Move to the initial point"
              # "current position"
              n116 = Array Size(array=w256) -> (size(s)=w255:i32)
              n117 = Bundle By Name(cluster=cluster{"Fs":dbl, "#s":dbl} {"Fs"=1000.0, "#s"=1000.0} ("sampling info"), "Fs"=w255, "#s"=w255) -> (w280:cluster{"Fs":dbl, "#s":dbl})
              n118 = call-poly <vilib>:"DAQmx Create Virtual Channel.vi"("maximum value"=10.0 ("Maximum Value 2"), "minimum value"=-10.0 ("Minimum Value 2"), "physical channels"="Starting Point for Scan") -> ("task out"=w286:refnum<k21>, "error out"=w285:errorcluster)  [unwired: 11 in]
              n119 = call <vilib>:"Basic Function Generator.vi"("offset"=w276, "sampling info"=w280, "signal type"=T1."Sawtooth Wave", "phase"=180.0, "amplitude"=w276, "frequency"=1.0) -> ("signal out"=w278:waveform(dbl))  [unwired: 3 in, 2 out]
              n120 = Index Array(array=w252, index (col)=0 ("disabled index (col)")) -> (element=w272:dbl[])  [unwired: 1 in]
              n121 = Unbundle By Name(w278) -> ("Y"=w258:dbl[])
              n122 = call-poly <vilib>:"DAQmx Read.vi"("task/channels in"=w286, "timeout"=10.0, "error in"=w285) -> ("data"=w274:dbl[])  [unwired: 10 in, 2 out]
              n123 = Index Array(array=w272, index=0) -> (element=w269:dbl)
              n124 = Index Array(array=w272, index=1) -> (element=w264:dbl)
              n125 = Index Array(array=w274, index=0) -> (element=w268:dbl)
              n126 = Index Array(array=w274, index=1) -> (element=w265:dbl)
              n127 = Subtract(x=w264, y=w265) -> (x-y=w263:dbl)
              n128 = Subtract(x=w269, y=w268) -> (x-y=w267:dbl)
              n129 = Multiply(x=w267, y=w258) -> (x*y=w266:dbl[])
              n130 = Multiply(x=w263, y=w258) -> (x*y=w262:dbl[])
              n131 = Add(x=w268, y=w266) -> (x+y=w261:dbl[])
              n132 = Add(x=w265, y=w262) -> (x+y=w260:dbl[])
              n133 = Divide(x=w247, y=2) -> (x/y=w250:dbl)
              n134 = Divide(x=w246, y=2) -> (x/y=w248:dbl)
              n135 = Build Array(w261, w260) -> (w253:dbl[][])
              n136 = property on="Channel2" class="IntensityGraph (strict)"("Cursor.Cursor Position:Cursor Y"=w248) -> ()  [unwired: 2 in, 2 out]
              n137 = property on="Channel2" class="IntensityGraph (strict)"("Cursor.Cursor Position:Cursor X"=w250) -> ()  [unwired: 2 in, 2 out]
              n138 = call-poly <vilib>:"DAQmx Write.vi"("task/channels in"=w254, "auto start"=TRUE, "data"=w253) -> ("task out"=w257:refnum<k21>)  [unwired: 10 in, 2 out]
              n139 = call <vilib>:"DAQmx Stop Task.vi"("task/channels in"=w257) -> ()  [unwired: 13 in, 2 out]
            }
            frame #4 {
              n140 = while {
                tunnel: w310 -> [w360]
                tunnel: w309 -> [w359]
                tunnel: w308 -> [w313]
                tunnel: [w341] -> w307
                tunnel: [w340] -> w306
                tunnel: [w338] -> w305
                tunnel: [w337] -> w304
                tunnel: [w336] -> w303
                tunnel: w302 -> [w335]
                tunnel: [w334] -> w301
                tunnel: w300 -> [w333]
                tunnel: w299 -> [w332]
                tunnel: w298 -> [w312]
                tunnel: [w331] -> w297
                tunnel: [w330] -> w296
                tunnel: w295 -> [w327]
                tunnel: [w326] -> w294
                tunnel: w293 -> [w325]
                tunnel: w292 -> [w323]
                tunnel: [w321] -> w291
                tunnel: [w320] -> w290
                stop <- w317 stop-if-true
                n141 = property class="DAQmx Timing"(reference=w360, error in=w359) -> (reference out=w358:refnum<k21>, error out=w357:errorcluster, "Sample Clock:Rate"=→"Input rate":dbl)
                n142 = property class="DAQmx Timing"(reference=w312, error in=w313) -> (reference out=w314:refnum<k21>, error out=w354:errorcluster, "Sample Clock:Rate"=→"Output rate":dbl)
                n143 = call "Get Terminal Name with Device Prefix.vi"("error in (no error)"=w357, "Local Terminal Name"="ai/StartTrigger" ("terminal"), "task/channels in"=w358) -> ("error out"=w347:errorcluster, "Terminal Name with Device Prefix"=w355:tag, "task out"=w348:refnum<k21>)  [unwired: 6 in]
                n144 = call-poly <vilib>:"DAQmx Trigger.vi"("task/channels in"=w314, "source"=w355, "error in"=w354) -> ("task out"=w353:refnum<k21>, "error out"=w352:errorcluster)  [unwired: 11 in]
                n145 = call-poly <vilib>:"DAQmx Write.vi"("task/channels in"=w353, "data"=w332, "timeout"=10.0 ("Wirite Timeout"), "error in"=w352) -> ("task out"=w350:refnum<k21>, "error out"=w349:errorcluster)  [unwired: 9 in, 1 out]
                n146 = call <vilib>:"DAQmx Start Task.vi"("task/channels in"=w350, "error in"=w349) -> ("task out"=w329:refnum<k21>, "error out"=w346:errorcluster)  [unwired: 12 in]
                n147 = call <vilib>:"Merge Errors.vi"("error in 2 (no error)"=w346, "error in 1 (no error)"=w347) -> ("error out"=w345:errorcluster)  [unwired: 5 in]
                n148 = call <vilib>:"DAQmx Start Task.vi"("task/channels in"=w348, "error in"=w345) -> ("task out"=w328:refnum<k21>, "error out"=w344:errorcluster)  [unwired: 12 in]
                n149 = Unbundle By Name(w327) -> ("Continuous \nScan"=w339:bool)
                n150 = call <vilib>:"DAQmx Start Task.vi"("task/channels in"=w325, "error in"=w323) -> ("task out"=w316:refnum<k21>, "error out"=w324:errorcluster)  [unwired: 12 in]
                n151 = while {
                  tunnel: w328 -> [w411]
                  tunnel: w344 -> [w410]
                  tunnel: w329 -> [w400]
                  tunnel: w333 -> [w402]
                  tunnel: w327 -> [w398]
                  tunnel: [w406] -> w343
                  shift-right: [w389] -> _
                  shift-left: w335 -> [w403]
                  tunnel: ["Stop"] -> w341
                  shift-right: [w388] -> _
                  shift-left: w335 -> [w395]
                  tunnel: [w389] -> w331
                  tunnel: [w388] -> w330
                  tunnel: ["Reset"] -> w326
                  tunnel: w316 -> [w386]
                  tunnel: w324 -> [w385]
                  tunnel: [w384] -> w322
                  tunnel: ["Reset"] -> w319
                  tunnel: ["Stop"] -> w311
                  tunnel: ["?"] -> w318
                  tunnel: [w374] -> _
                  i -> [w383]
                  stop <- w412 stop-if-true
                  n152 = Unbundle By Name(w398) -> ("Scan Rate (Hz)"=w396:dbl, "Scan Lines"=w378:u32, "Continuous \nScan"=w397:bool, "Scan Points"=w392:u32, "Lines read"=w382:u32, "Scanner delay (ms)"=w394:dbl)
                  n153 = Quotient & Remainder(x=w402, y=w396) -> (floor(x/y)=w399:dbl)  [unwired: 1 out]
                  n154 = Multiply(x=w399, y=w382) -> (x*y=w390:dbl)
                  n155 = call-poly <vilib>:"DAQmx Read.vi"("task/channels in"=w411, "number of samples per channel"=w390, "error in"=w410) -> ("data"=w381:dbl[][], "error out"=w409:errorcluster)  [unwired: 10 in, 1 out]
                  n156 = call <vilib>:"DAQmx Is Task Done.vi"("task/channels in"=w400, "error in"=w409) -> ("task out"=w374:refnum<k21>, "error out"=w408:errorcluster)  [unwired: 11 in, 1 out]
                  n157 = Unbundle By Name(w408) -> ("status"=w407:bool)
                  n158 = call <vilib>:"DAQmx Is Read or Write Late.vi"("error in"=w408) -> ("error out"=w406:errorcluster)  [unwired: 13 in, 1 out]
                  n159 = Quotient & Remainder(x=w378, y=w382) -> (floor(x/y)=w391:u32)  [unwired: 1 out]
                  n160 = Compound Arithmetic op=MULTIPLY(w394, w402, 0.001 ("value")) -> (w371:dbl)
                  n161 = Greater Or Equal?(x=w383, y=w391) -> (x >= y?=w405:bool)
                  n162 = stacked-sequence {
                    seq-local: [w448 _] -> [_ w540]
                    tunnel: w403 -> [w455 w541]
                    tunnel: [w445 _] -> w389
                    tunnel: w371 -> [w454 _]
                    tunnel: w383 -> [w453 _]
                    tunnel: w392 -> [w452 _]
                    tunnel: w399 -> [w451 _]
                    tunnel: w378 -> [w447 _]
                    tunnel: w381 -> [w450 _]
                    tunnel: w382 -> [w444 _]
                    tunnel: w395 -> [w449 w535]
                    tunnel: [w446 _] -> w388
                    tunnel: [_ w536] -> w393
                    frame #0 {
                      n163 = while {
                        tunnel: w450 -> [w481]
                        tunnel: w453 -> [w465]
                        tunnel: w447 -> [w469]
                        tunnel: w451 -> [w476]
                        tunnel: w452 -> [w473]
                        tunnel: w444 -> [w466]
                        shift-right: [w479] -> w445
                        shift-left: w455 -> [w480]
                        tunnel: w454 -> [w461]
                        tunnel: [w456] -> w443
                        i -> [w463]
                        stop <- w471 stop-if-true
                        n164 = Decrement(x=w466) -> (x-1=w472:u32)
                        n165 = Index Array(array=w481, index (row)=0) -> (element=w478:dbl[])  [unwired: 1 in]
                        n166 = Multiply(x=w465, y=w466) -> (x*y=w467:u32)
                        n167 = Add(x=0.26666 ("value"), y=w463) -> (x+y=w459:dbl)
                        n168 = Greater Or Equal?(x=w463, y=w472) -> (x >= y?=w471:bool)
                        n169 = Add(x=w467, y=w463) -> (x+y=w468:u32)
                        n170 = Compound Arithmetic op=MULTIPLY(w459, w476) -> (w462:dbl)
                        n171 = Quotient & Remainder(x=w468, y=w469) -> (x-y*floor(x/y)=w470:u32)  [unwired: 1 out]
                        n172 = Add(x=w461, y=w462) -> (x+y=w460:dbl)
                        n173 = Negate(x=w460) -> (-x=w458:dbl)
                        n174 = Round To Nearest(number=w458) -> (nearest integer value=w477:dbl)
                        n175 = Rotate 1D Array(1:w478, 2:w477) -> (0:w457:dbl[])
                        n176 = Initialize Array(0.0 ("element"), w473) -> (w475:dbl[])
                        n177 = while {
                          tunnel: w457 -> [w491]
                          tunnel: w473 -> [w488]
                          tunnel: w476 -> [w493]
                          shift-right: [w486] -> w456
                          shift-left: w475 -> [w485]
                          i -> [w483]
                          stop <- w489 stop-if-true
                          n178 = Decrement(x=w488) -> (x-1=w487:u32)
                          n179 = Greater Or Equal?(x=w483, y=w487) -> (x >= y?=w489:bool)
                          n180 = Compound Arithmetic op=MULTIPLY(0.6666 ("value"), w493, w483) -> (w492:dbl)
                          n181 = Quotient & Remainder(x=w492, y=w488) -> (floor(x/y)=w490:dbl)  [unwired: 1 out]
                          n182 = Index Array(array=w491, index=w490) -> (element=w484:dbl)
                          n183 = Replace Array Subset(array=w485, new element=w484, index=w483) -> (w486:dbl[])
                        }
                        n184 = Replace Array Subset(array=w480, new element=w456, index (col)=w470) -> (w479:dbl[][])  [unwired: 1 in]
                      }
                      "Reflection Image" <- w445
                      n185 = while {
                        tunnel: w450 -> [w520]
                        tunnel: w453 -> [w507]
                        tunnel: w447 -> [w510]
                        tunnel: w451 -> [w515]
                        tunnel: w452 -> [w512]
                        tunnel: w444 -> [w497]
                        shift-right: [w518] -> w446
                        shift-left: w449 -> [w519]
                        tunnel: w454 -> [w504]
                        tunnel: [w496] -> w448
                        tunnel: [w495] -> w442
                        i -> [w498]
                        stop <- w499 stop-if-true
                        n186 = Decrement(x=w497) -> (x-1=w511:u32)
                        n187 = Index Array(array=w520, index (row)=1) -> (element=w517:dbl[])  [unwired: 1 in]
                        n188 = Multiply(x=w507, y=w497) -> (x*y=w508:u32)
                        n189 = Add(x=0.26666 ("value"), y=w498) -> (x+y=w502:dbl)
                        n190 = Greater Or Equal?(x=w498, y=w511) -> (x >= y?=w499:bool)
                        n191 = Add(x=w508, y=w498) -> (x+y=w509:u32)
                        n192 = Compound Arithmetic op=MULTIPLY(w502, w515) -> (w505:dbl)
                        n193 = Quotient & Remainder(x=w509, y=w510) -> (x-y*floor(x/y)=w496:u32)  [unwired: 1 out]
                        n194 = Add(x=w504, y=w505) -> (x+y=w503:dbl)
                        n195 = Negate(x=w503) -> (-x=w501:dbl)
                        n196 = Round To Nearest(number=w501) -> (nearest integer value=w516:dbl)
                        n197 = Rotate 1D Array(1:w517, 2:w516) -> (0:w500:dbl[])
                        n198 = Initialize Array(0.0 ("element"), w512) -> (w514:dbl[])
                        n199 = while {
                          tunnel: w500 -> [w530]
                          tunnel: w512 -> [w527]
                          tunnel: w515 -> [w532]
                          shift-right: [w525] -> w495
                          shift-left: w514 -> [w524]
                          i -> [w522]
                          stop <- w528 stop-if-true
                          n200 = Decrement(x=w527) -> (x-1=w526:u32)
                          n201 = Greater Or Equal?(x=w522, y=w526) -> (x >= y?=w528:bool)
                          n202 = Compound Arithmetic op=MULTIPLY(0.6666 ("value"), w532, w522) -> (w531:dbl)
                          n203 = Quotient & Remainder(x=w531, y=w527) -> (floor(x/y)=w529:dbl)  [unwired: 1 out]
                          n204 = Index Array(array=w530, index=w529) -> (element=w523:dbl)
                          n205 = Replace Array Subset(array=w524, new element=w523, index=w522) -> (w525:dbl[])
                        }
                        n206 = Replace Array Subset(array=w519, new element=w495, index (col)=w496) -> (w518:dbl[][])  [unwired: 1 in]
                      }
                      "Channel2" <- w446
                      n207 = Build Array(w443, w442) -> (→"Linescan":dbl[][])
                    }
                    frame #1 {
                      n208 = property on="Scan Lines" class="Digital (strict)"() -> ("Value"=w538:u32)  [unwired: 2 in, 2 out]
                      n209 = Decrement(x=w538) -> (x-1=w537:u32)
                      n210 = Equal?(x=w537, y=w540) -> (x = y?=w539:bool)
                      n211 = And(x="Save Image", y=w539) -> (x .and. y?=w536:bool)
                      n212 = case shown="True" w536 {
                        tunnel: w541 -> [_ w555]
                        tunnel: w535 -> [_ w554]
                        frame #0 {
                        }
                        frame #1 {
                          w557 = "%.3f" ("format string")
                          w560 = T3."create or replace" ("function (open:0)")
                          n213 = case shown="True" "Concat" {
                            tunnel: [w570 w573] -> w548
                            tunnel: "Channel 2" -> [w570 w574]
                            tunnel: [w569 w580] -> w546
                            tunnel: "Channel 1" -> [w569 w585]
                            frame #0 {
                            }
                            frame #1 {
                              w572 = "_"
                              n214 = local read "Output4"() -> (w582:dbl)
                              n215 = Multiply(x=w582, y=1000) -> (x*y=w581:dbl)
                              n216 = Strip Path(path=w585) -> (stripped path=w579:path, name=w584:string)
                              n217 = Strip Path(path=w574) -> (stripped path=w576:path, name=w577:string)
                              n218 = Number To Decimal String(number=w581) -> (decimal integer string=w571:string)  [unwired: 1 in]
                              n219 = Concatenate Strings(w584, w572, w571) -> (w578:string)
                              n220 = Concatenate Strings(w577, w572, w571) -> (w575:string)
                              n221 = Build Path(base path=w579, name or relative path=w578) -> (appended path=w580:path)
                              n222 = Build Path(base path=w576, name or relative path=w575) -> (appended path=w573:path)
                            }
                          }
                          n223 = call <vilib>:"Open_Create_Replace File.vi"("function (open:0)"=w560, "file path"=w546) -> ("error out"=w566:errorcluster, "refnum"=w568:refnum<file>)  [unwired: 6 in, 2 out]
                          n224 = call <vilib>:"Open_Create_Replace File.vi"("function (open:0)"=w560, "file path"=w548) -> ("error out"=w564:errorcluster, "refnum"=w563:refnum<file>)  [unwired: 6 in, 2 out]
                          n225 = Array To Spreadsheet String(array=w554, 3:w557) -> (spreadsheet string=w558:string)  [unwired: 1 in]
                          n226 = Array To Spreadsheet String(array=w555, 3:w557) -> (spreadsheet string=w559:string)  [unwired: 1 in]
                          n227 = Write to Binary File(file (use dialog)=w563, data=w558, error in=w564, 5:FALSE ("prepend array or string size? (T)")) -> (refnum out=w562:refnum<file>, error out=w561:errorcluster)  [unwired: 2 in, 1 out]
                          n228 = Write to Binary File(file (use dialog)=w568, data=w559, error in=w566, 5:FALSE ("prepend array or string size? (T)")) -> (refnum out=w567:refnum<file>, error out=w565:errorcluster)  [unwired: 2 in, 1 out]
                          n229 = property on="Increment" class="Bool (strict)"() -> ("Value"=w549:bool)  [unwired: 2 in, 2 out]
                          n230 = Close File(refnum=w567, error in=w565) -> (error out=w556:errorcluster)  [unwired: 1 out]
                          n231 = Close File(refnum=w562, error in=w561) -> (error out=w552:errorcluster)  [unwired: 1 out]
                          n232 = call <vilib>:"Merge Errors.vi"("error in 2 (no error)"=w552, "error in 1 (no error)"=w556) -> ("error out"=w553:errorcluster)  [unwired: 5 in]
                          n233 = call <vilib>:"Simple Error Handler.vi"("error in (no error)"=w553) -> ("error?"=w550:bool)  [unwired: 4 in, 4 out]
                          n234 = Or(x=w550, y=w549) -> (x .or. y?=w551:bool)
                          n235 = local write "Save Image"(w551) -> ()
                        }
                      }
                    }
                  }
                  n236 = Not(x=w397) -> (.not. x?=w404:bool)
                  n237 = And(x=w405, y=w404) -> (x .and. y?=w387:bool)
                  n238 = Multiply(x=w383, y=w382) -> (x*y=w379:u32)
                  n239 = Divide(x=w379, y=w378) -> (x/y=w377:dbl)
                  n240 = Quotient & Remainder(x=w379, y=w378) -> (floor(x/y)=w380:u32)  [unwired: 1 out]
                  n241 = Equal?(x=w380, y=w377) -> (x = y?=w373:bool)
                  n242 = And(x="Increment", y=w373) -> (x .and. y?=w368:bool)
                  n243 = case shown="True" w368 {
                    tunnel: "Output4" -> [w427 w428]
                    tunnel: [w427 w429] -> w367
                    frame #0 {
                    }
                    frame #1 {
                      n244 = Greater?(x="stepsize", y=0) -> (0:w433:bool)
                      n245 = Less?(x=w428, y="StopPoint") -> (x < y?=w432:bool)
                      n246 = Exclusive Or(1:w432, 2:w433) -> (0:w431:bool)
                      n247 = case shown="True" w431 {
                        tunnel: "stepsize" -> [w438 _]
                        tunnel: w428 -> [w437 w439]
                        tunnel: [w436 w439] -> w429
                        frame #0 {
                          n248 = Add(x=w437, y=w438) -> (x+y=w436:dbl)
                        }
                        frame #1 {
                          n249 = local write "Increment"(FALSE) -> ()
                        }
                      }
                    }
                  }
                  n250 = event shown="[2] \"Channel2\": Mouse Enter" {
                    selector: _ -> [_ _ _]
                    dyn-events: _ -> [_ _ _]
                    timeout: 0 -> [_ _ _]
                    tunnel: [w413 TRUE FALSE] -> w366
                    event #0 {
                      n251 = event-data() -> ()  [unwired: 1 in, 2 out]
                      n252 = local read "Boolean"() -> (w413:bool)
                    }
                    event #1 {
                      n253 = event-data() -> ()  [unwired: 1 in, 4 out]
                    }
                    event #2 {
                      n254 = event-data() -> ()  [unwired: 1 in, 4 out]
                    }
                  }
                  "Boolean" <- w366
                  n255 = Compound Arithmetic op=OR(w387, "Reset", "Stop", w407, w393, "?", "?") -> (w412:bool)
                  n256 = case shown="False" w366 {
                    frame #0 {
                      n257 = property on="Channel2" class="IntensityGraph (strict)"() -> ("Cursor.Cursor Position"=w416:T4)  [unwired: 2 in, 2 out]
                      n258 = property on="Reflection Image" class="IntensityGraph (strict)"("Cursor.Cursor Position"=w416) -> ()  [unwired: 2 in, 2 out]
                    }
                    frame #1 {
                      n259 = property on="Reflection Image" class="IntensityGraph (strict)"() -> ("Cursor.Cursor Position"=w417:T4)  [unwired: 2 in, 2 out]
                      n260 = property on="Channel2" class="IntensityGraph (strict)"("Cursor.Cursor Position"=w417) -> ()  [unwired: 2 in, 2 out]
                    }
                  }
                  n261 = local write "Output4"(w367) -> ()
                  n262 = Or(x=w368, y="Update") -> (x .or. y?=w370:bool)
                  n263 = case shown="True" w370 {
                    tunnel: w386 -> [_ w426]
                    tunnel: w385 -> [w418 w423]
                    tunnel: [w418 w422] -> w384
                    tunnel: w367 -> [_ w419]
                    frame #0 {
                    }
                    frame #1 {
                      n264 = Bundle("Output4"=w419, "Output3"="Output3") -> (w424:cluster{"Output4":dbl, "Output3":dbl})  [unwired: 1 in]
                      n265 = local write "Update"(FALSE ("Update")) -> ()
                      n266 = Cluster To Array(cluster=w424) -> (array=w425:dbl[])
                      n267 = call-poly <vilib>:"DAQmx Write.vi"("task/channels in"=w426, "data"=w425, "error in"=w423) -> ("error out"=w422:errorcluster)  [unwired: 10 in, 2 out]
                    }
                  }
                }
                n268 = Not(x=w339) -> (.not. x?=w334:bool)
                n269 = call <vilib>:"DAQmx Stop Task.vi"("task/channels in"=w329, "error in"=w343) -> ("task out"=w336:refnum<k21>, "error out"=w342:errorcluster)  [unwired: 12 in]
                n270 = call <vilib>:"DAQmx Stop Task.vi"("task/channels in"=w328, "error in"=w342) -> ("task out"=w338:refnum<k21>, "error out"=w337:errorcluster)  [unwired: 12 in]
                n271 = Unbundle By Name(w337) -> ("status"=w340:bool)
                n272 = case shown="True" w318 {
                  frame #0 {
                  }
                  frame #1 {
                    n273 = while {
                      stop <- w362 continue-if-true
                      n274 = property class="Boolean (strict)"() -> ("Value"=w362:bool)  [unwired: 2 in, 2 out]
                    }
                  }
                }
                n275 = call <vilib>:"DAQmx Stop Task.vi"("task/channels in"=w316, "error in"=w322) -> ("task out"=w320:refnum<k21>, "error out"=w321:errorcluster)  [unwired: 12 in]
                n276 = Compound Arithmetic op=OR(w319, w311) -> (w317:bool)
              }
            }
            frame #5 {
              n277 = property on="Channel2" class="IntensityGraph (strict)"() -> ("Cursor.Cursor Position"=w591:T4)  [unwired: 2 in, 2 out]
              n278 = Bundle("Value"=w586, "Value"=w587) -> (w606:cluster{"Value":u32, "Value":u32})  [unwired: 1 in]
              n279 = Unbundle By Name(w612) -> ("Scan Angle (degrees)"=w615:dbl)
              n280 = Reciprocal(x=180.0 ("value")) -> (1/x=w613:dbl)
              n281 = Divide(x=w606, y=2) -> (x/y=w611:cluster{"Value":dbl, "Value":dbl})
              n282 = Compound Arithmetic op=MULTIPLY(w615, w613, 3.141592653589793) -> (w616:dbl)
              n283 = Subtract(x=w591, y=w611) -> (x-y=w607:T4)
              n284 = Sine & Cosine(0:w616) -> (1:w610:dbl, 2:w609:dbl)
              n285 = Divide(x=w607, y=w606) -> (x/y=w608:T4)
              n286 = Negate(x=w610) -> (-x=w588:dbl)
              n287 = Multiply(x=w588, y=w608) -> (x*y=w604:T4)
              n288 = Multiply(x=w609, y=w608) -> (x*y=w605:T4)
              n289 = Unbundle(w605) -> ("Cursor X"=w603:dbl, "Cursor Y"=w601:dbl)
              n290 = Unbundle(w604) -> ("Cursor X"=w600:dbl, "Cursor Y"=w602:dbl)
              n291 = property on="Y Scan size(um)" class="Digital (strict)"() -> ("Value"=w597:dbl)  [unwired: 2 in, 2 out]
              n292 = Negate(x=w600) -> (-x=w599:dbl)
              n293 = Add(x=w602, y=w603) -> (x+y=w592:dbl)
              n294 = Add(x=w599, y=w601) -> (x+y=w590:dbl)
              n295 = property on="X Scan size(um)" class="Digital (strict)"() -> ("Value"=w598:dbl)  [unwired: 2 in, 2 out]
              n296 = Negate(x=w597) -> (-x=w589:dbl)
              n297 = Bundle(w592, w590) -> (w596:cluster{dbl, dbl})  [unwired: 1 in]
              n298 = Bundle("Value"=w598, w589) -> (w595:cluster{"Value":dbl, dbl})  [unwired: 1 in]
              n299 = Multiply(x=w596, y=w595) -> (x*y=w593:cluster{dbl, dbl})
              n300 = flat-sequence {
                tunnel: [w621] -> w594
                tunnel: w594 -> [w626]
                tunnel: w593 -> [w625]
                frame #0 {
                  n301 = local read "Y offset (um)"() -> (w619:dbl)
                  n302 = local read "X offset (um)"() -> (w620:dbl)
                  n303 = Bundle("X offset (um)"=w620, "Y offset (um)"=w619) -> (w621:T5)  [unwired: 1 in]
                }
                frame #1 {
                  n304 = Subtract(x=w626, y=w625) -> (x-y=w624:cluster{dbl, dbl})
                  n305 = Unbundle(w624) -> (w623:dbl, w622:dbl)
                  n306 = local write "Y offset (um)"(w622) -> ()
                  n307 = local write "X offset (um)"(w623) -> ()
                }
              }
            }
          }
          n308 = Compound Arithmetic op=OR(w77, w81, w89, w76) -> (w86:bool)
        }
        n309 = call <vilib>:"DAQmx Clear Task.vi"("task in"=w52, "error in"=w53) -> ()  [unwired: 13 in, 1 out]
        n310 = call <vilib>:"DAQmx Clear Task.vi"("task in"=w66, "error in"=w65) -> ("error out"=w54:errorcluster)  [unwired: 13 in]
        n311 = call <vilib>:"DAQmx Clear Task.vi"("task in"=w64, "error in"=w54) -> ("error out"=w63:errorcluster)  [unwired: 13 in]
        n312 = call <vilib>:"General Error Handler.vi"("error in (no error)"=w63) -> ()  [unwired: 10 in, 5 out]
      }
    }
  }
